vi "SortZtoATest.vi"(11 "error in":errorcluster) -> (15 "error out":errorcluster)   [LabVIEW 2023, in "TestVIs.lvlib"]
uses:
  TestVIs.lvlib
  <vilib>/SLL Toolkit/SLL String/_SubVIs/1D String Array to String.vi
  <vilib>/addons/_JKI Toolkits/Caraya/classes/Assert/Assert Equal Value_Variant.vi
  <vilib>/addons/_JKI Toolkits/Caraya/classes/Test/Test.lvclass
  <vilib>/addons/_JKI Toolkits/Caraya/classes/Assert/Assert.lvclass
  Library/Unit Testing CA1.lvlib
  <vilib>/SLL Toolkit/SLL String/SLL String.lvlib
panel:
  # "REVERSE SORT TEST"
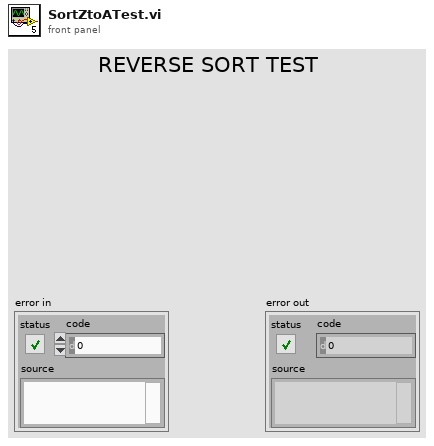
[diagram p1: front panel]
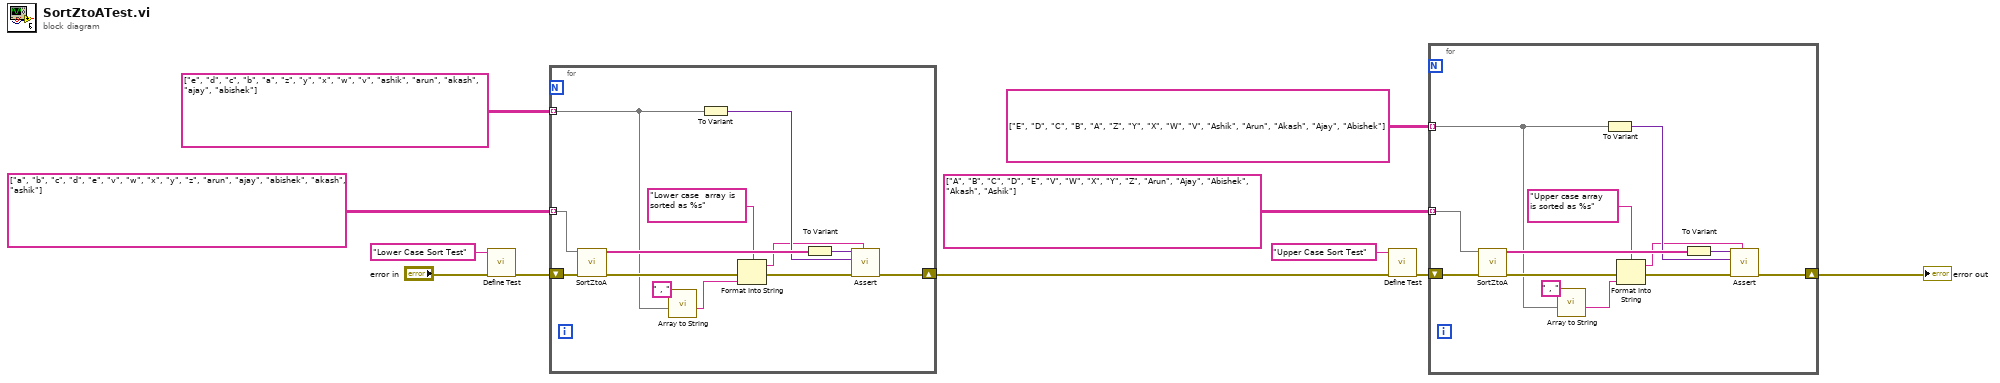
[diagram p0: block diagram]
diagram:
  n1 = call <vilib>:"Define Test.vi"("error in (no error)"="error in", "Label (VI Title)"="Lower Case Sort Test") -> ("error out"=w9:errorcluster)  [unwired: 8 in, 1 out]
  n2 = for {
    shift-right: [w17] -> w2
    shift-left: w9 -> [w24]
    tunnel: string[][] [["a", "b", "c", "d", "e"], ["v", "w", "x", "y", "z"], ["arun", "ajay", "abishek", "akash", "ashik"]] ("Input Array") -> [w16] mode=indexing
    tunnel: string[][] [["e", "d", "c", "b", "a"], ["z", "y", "x", "w", "v"], ["ashik", "arun", "akash", "ajay", "abishek"]] ("Input Array") -> [w15] mode=indexing
    n3 = call "SortZtoA.vi"("Input Array"=w16, "error in"=w24) -> ("reversed array"=w23:string[], "error out"=w20:errorcluster)  [unwired: 12 in]
    n4 = call-poly <vilib>:"Array to String.vi"("Delimiter (,)"=" , ", "1D Array[]"=w15) -> ("String"=w14:string)  [unwired: 6 in]
    n5 = To Variant(anything=w15) -> (Variant=w22:variant)
    n6 = Format Into String(format string="Lower case  array is sorted as %s", error in=w20, w14) -> (resulting string=w18:string, error out=w19:errorcluster)  [unwired: 1 in]
    n7 = To Variant(anything=w23) -> (Variant=w21:variant)
    n8 = call-poly <vilib>:"Assert.vi"("Label"=w18, "error in (no error)"=w19, "Y"=w22, "X"=w21) -> ("error out"=w17:errorcluster)  [unwired: 6 in, 1 out]
  }
  n9 = call <vilib>:"Define Test.vi"("error in (no error)"=w2, "Label (VI Title)"="Upper Case Sort Test") -> ("error out"=w5:errorcluster)  [unwired: 8 in, 1 out]
  n10 = for {
    shift-right: [w30] -> w1
    shift-left: w5 -> [w37]
    tunnel: string[][] [["A", "B", "C", "D", "E"], ["V", "W", "X", "Y", "Z"], ["Arun", "Ajay", "Abishek", "Akash", "Ashik"]] ("Input Array") -> [w29] mode=indexing
    tunnel: string[][] [["E", "D", "C", "B", "A"], ["Z", "Y", "X", "W", "V"], ["Ashik", "Arun", "Akash", "Ajay", "Abishek"]] ("Input Array") -> [w27] mode=indexing
    n11 = call "SortZtoA.vi"("Input Array"=w29, "error in"=w37) -> ("reversed array"=w36:string[], "error out"=w33:errorcluster)  [unwired: 12 in]
    n12 = call-poly <vilib>:"Array to String.vi"("Delimiter (,)"=" , ", "1D Array[]"=w27) -> ("String"=w26:string)  [unwired: 6 in]
    n13 = To Variant(anything=w27) -> (Variant=w35:variant)
    n14 = Format Into String(format string="Upper case array is sorted as %s", error in=w33, w26) -> (resulting string=w31:string, error out=w32:errorcluster)  [unwired: 1 in]
    n15 = To Variant(anything=w36) -> (Variant=w34:variant)
    n16 = call-poly <vilib>:"Assert.vi"("Label"=w31, "error in (no error)"=w32, "Y"=w35, "X"=w34) -> ("error out"=w30:errorcluster)  [unwired: 6 in, 1 out]
  }
  "error out" <- w1
